vi "4.1.vi"() -> ()   [LabVIEW 2016]
panel:
  out "数组":dbl[](array[numeric])
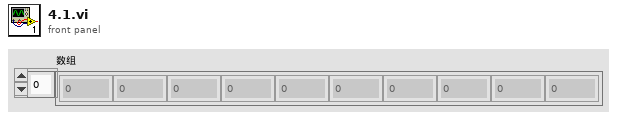
[diagram p1: front panel]
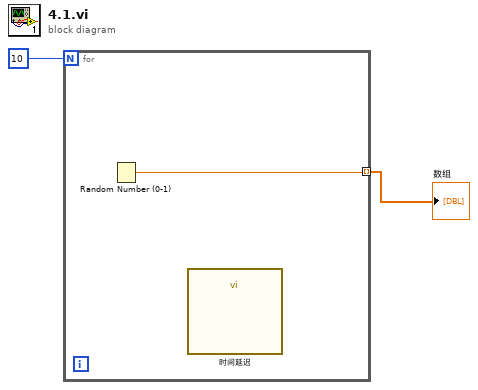
[diagram p0: block diagram]
diagram:
  n1 = for {
    N: 10 -> [_]
    tunnel: [w3] -> w1 mode=indexing
    n2 = Random Number (0-1)() -> (number: 0 to 1=w3:dbl)
    n3 = call "时间延迟"() -> ()  [unwired: 11 in, 1 out]
  }
  "数组" <- w1
